vi "config_file.vi"(8 "error in":errorcluster, 11 "reference cluster in":T1) -> (0 "error out":errorcluster, 3 "reference cluster out":T1)   [LabVIEW 2016]
uses:
  Type Definitions/reference_cluster.ctl
  Type Definitions/vars_settings.ctl
  Type Definitions/stim_type.ctl
  Type Definitions/vars_runtime.ctl
  Type Definitions/data.ctl
  Type Definitions/notifier_elements_GUI.ctl
  Type Definitions/notifier_elements_DAQ.ctl
  Type Definitions/notifier_elements_write.ctl
  Type Definitions/control_references.ctl
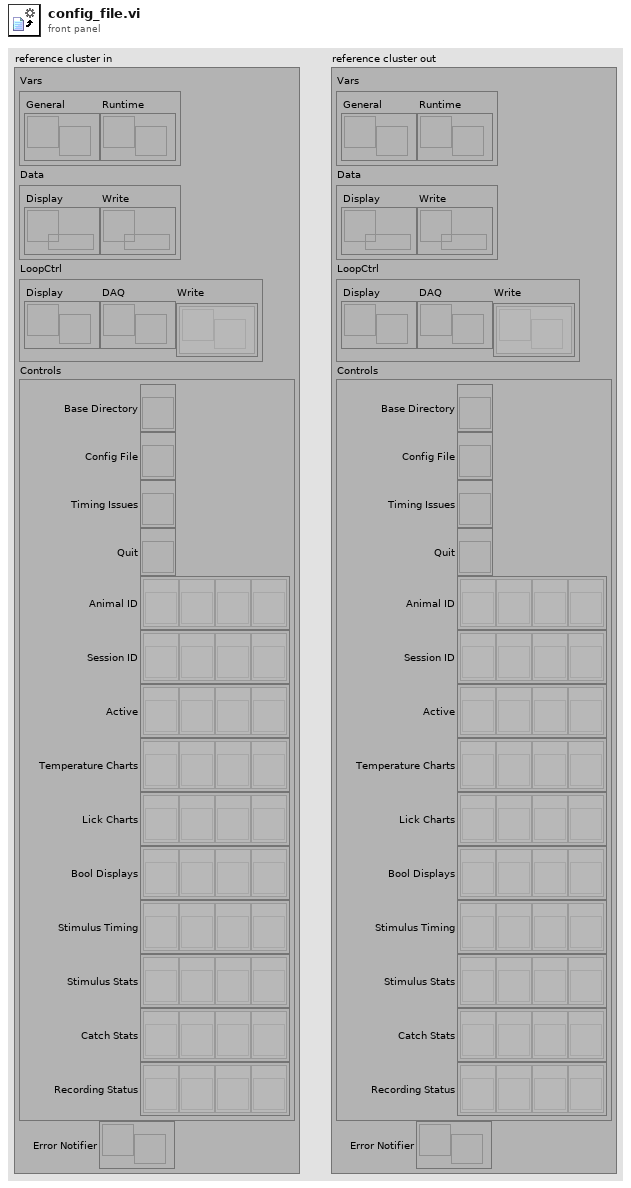
[diagram p1: front panel]
types:
  T1 = typedef "reference_cluster.ctl" = cluster{"Vars":cluster{"General":refnum<notifier>, "Runtime":refnum<notifier>}, "Data":cluster{"Display":refnum<queue>, "Write":refnum<queue>}, "LoopCtrl":cluster{"Display":refnum<notifier>, "DAQ":refnum<notifier>, "Write":refnum<notifier>[]}, "Controls":T2, "Error Notifier":refnum<notifier>}
  T2 = typedef "control_references.ctl" = cluster{"Base Directory":refnum<vi>, "Config File":refnum<vi>, "Timing Issues":refnum<vi>, "Quit":refnum<vi>, "Animal ID":refnum<vi>[], "Session ID":refnum<vi>[], "Active":refnum<vi>[], "Temperature Charts":refnum<vi>[], "Lick Charts":refnum<vi>[], "Bool Displays":refnum<vi>[], "Stimulus Timing":refnum<vi>[], "Stimulus Stats":refnum<vi>[], "Catch Stats":refnum<vi>[], "Recording Status":refnum<vi>[]}
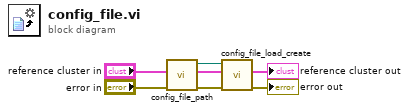
[diagram p0: block diagram]
diagram:
  n1 = call "config_file_path.vi"("error in"="error in", "reference cluster in"="reference cluster in") -> ("error out"=w4:errorcluster, "reference cluster out"=w3:T1, "path"=w2:path)  [unwired: 7 in]
  n2 = call "config_file_load_create.vi"("configuration file path"=w2, "reference cluster in"=w3, "error in"=w4) -> ("reference cluster out"=→"reference cluster out":T1, "error out"=→"error out":errorcluster)  [unwired: 6 in]
